vi "enableDisable.vi"(8 "error in (no error)":errorcluster, 10 "Controls - Status":T1(array[cluster]), 11 "uiControlsMgr in":refnum<class "uiControlsMgr.lvclass">=refnum) -> (0 "error out":errorcluster, 3 "uiControlsMgr out":refnum<class "uiControlsMgr.lvclass">)   [LabVIEW 2020, in "UI Controls Manager.lvlib" / "uiControlsMgr.lvclass"]
uses:
  uiControlsMgr.lvclass
  uiControlsMgr.lvclass/uiControlsMgr.ctl
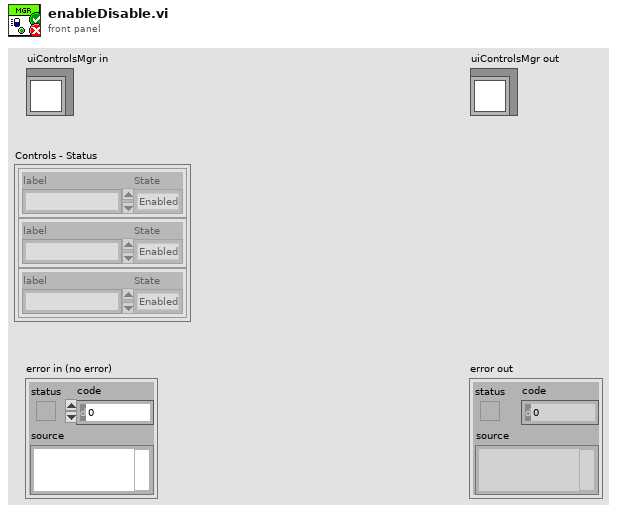
[diagram p1: front panel]
types:
  T1 = cluster{"label":string, "State":enum8{"Enabled", "Disabled", "Disabled and Grayed Out"}}[]
  T2 = map{string, cluster{"Caption":string, "Ctl Refnum":refnum<vi>}}
  T3 = enum8{"Enabled", "Disabled", "Disabled and Grayed Out"}
  T4 = cluster{"Caption":string, "Ctl Refnum":refnum<vi>}
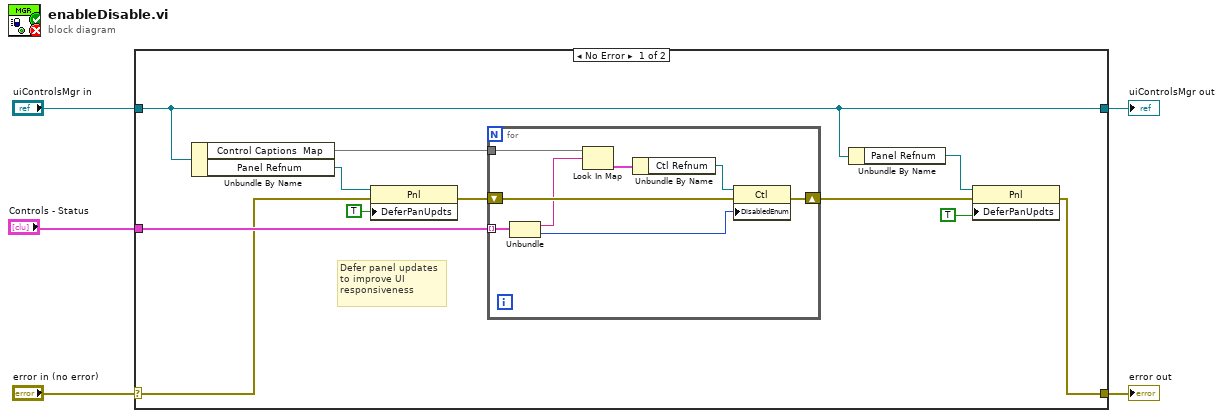
[diagram p0: block diagram]
diagram:
  n1 = case shown="No Error" "error in (no error)" {
    selector: "error in (no error)" -> [w7 w26]
    tunnel: [w6 w26] -> w4
    tunnel: [w9 w25] -> w2
    tunnel: "uiControlsMgr in" -> [w9 w25]
    tunnel: "Controls - Status" -> [w15 _]
    frame No Error {
      # "Defer panel updates\nto improve UI\nresponsiveness"
      n2 = Unbundle By Name(w9) -> ("Control Captions  Map"=w16:T2, "Panel Refnum"=w14:refnum<vi>)
      n3 = property class="Pnl"(reference=w14, error in=w7, "DeferPanUpdts"=TRUE ("Defer Panel Updates")) -> (error out=w12:errorcluster)  [unwired: 1 out]
      n4 = for {
        tunnel: w16 -> [w24]
        tunnel: w15 -> [w19] mode=indexing
        shift-right: [w20] -> w10
        shift-left: w12 -> [w21]
        n5 = Unbundle(w19) -> ("label"=w18:string, "State"=w17:T3)
        n6 = Look In Map(map=w24, key=w18) -> (value=w23:T4)  [unwired: 1 in, 1 out]
        n7 = Unbundle By Name(w23) -> ("Ctl Refnum"=w22:refnum<vi>)
        n8 = property class="Ctl"(reference=w22, error in=w21, "DisabledEnum"=w17) -> (error out=w20:errorcluster)  [unwired: 1 out]
      }
      n9 = Unbundle By Name(w9) -> ("Panel Refnum"=w8:refnum<vi>)
      n10 = property class="Pnl"(reference=w8, error in=w10, "DeferPanUpdts"=TRUE ("Defer Panel Updates")) -> (error out=w6:errorcluster)  [unwired: 1 out]
    }
    frame Error {
    }
  }
  "error out" <- w4
  "uiControlsMgr out" <- w2
